vi "GET_MARKER.vi"(5 "offset":dbl, 6 "Set MKR Freq (MHz)":dbl=2000000.0 format="%#_13g", 7 "Use PK Search (T)":bool=TRUE, 8 "error in":errorcluster {"code" format="%.0x"}, 11 "Session In":refnum<visa-resource-name>="TCPIP0::169.254.70.120::inst0::INSTR") -> (0 "error out":errorcluster {"code" format="%.0x"}, 1 "Ampl_corr":dbl=-76.918, 2 "Mark Values":dbl[](array[numeric])=[40000.0232, -76.918], 3 "Session Out":refnum<visa-resource-name>="TCPIP0::169.254.70.120::inst0::INSTR")   [LabVIEW 2018]
doc: "Launches the Instrument I/O Assistant, which you can use to communicate with message-based instruments and graphically parse the response. For example you can communicate with an instrument that uses a serial, Ethernet, or GPIB interface."
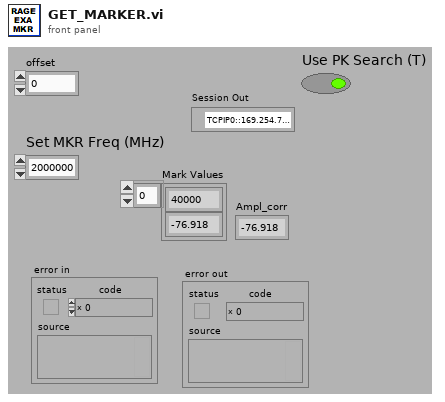
[diagram p1: front panel]
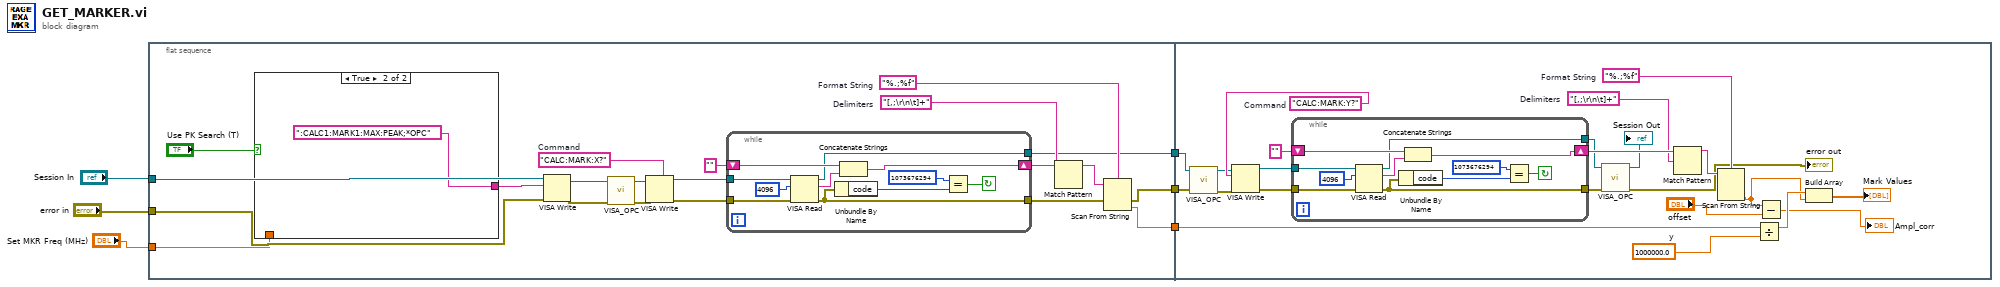
[diagram p0: block diagram]
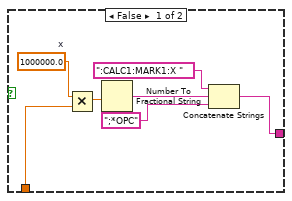
[diagram p2: hidden frame]
diagram:
  n1 = flat-sequence {
    tunnel: [w20] -> w6
    tunnel: "error in" -> [w19]
    tunnel: "Session In" -> [w18]
    tunnel: [w17] -> w4
    tunnel: [w16] -> w2
    tunnel: "Set MKR Freq (MHz)" -> [w13]
    tunnel: w6 -> [w54]
    tunnel: w4 -> [w52]
    tunnel: w2 -> [w60]
    frame #0 {
      w21 = "[,;\r\n\t]+"  # Delimiters
      w22 = "%.;%f"  # Format String
      w25 = "CALC:MARK:X?"  # Command
      n2 = case shown="True" "Use PK Search (T)" {
        tunnel: [w29 ":CALC1:MARK1:MAX:PEAK;*OPC" ("StaticText")] -> w15
        tunnel: w13 -> [w28 _]
        frame False {
          w32 = 1000000.0  # x
          n3 = Multiply(x=w32, y=w28) -> (x*y=w34:dbl)
          n4 = Number To Fractional String(number=w34) -> (F-format string=w33:string)  [unwired: 3 in]
          n5 = Concatenate Strings(":CALC1:MARK1:X " ("StaticText"), w33, ";*OPC" ("string")) -> (w29:string)
        }
        frame True {
        }
      }
      n6 = VISA Write(VISA resource name=w18, write buffer=w15, error in (no error)=w19) -> (VISA resource name out=w10:refnum<visa-resource-name>, error out=w11:errorcluster)  [unwired: 1 out]
      n7 = call "VISA_OPC.vi"("error in"=w11, "Session In"=w10) -> ("error out"=w12:errorcluster, "Session Out"=w9:refnum<visa-resource-name>)  [unwired: 7 in, 1 out]
      n8 = VISA Write(VISA resource name=w9, write buffer=w25, error in (no error)=w12) -> (VISA resource name out=w8:refnum<visa-resource-name>, error out=w7:errorcluster)  [unwired: 1 out]
      n9 = while {
        tunnel: w8 -> [w43]
        shift-right: [w37] -> w24
        shift-left: "" -> [w42]
        tunnel: w7 -> [w40]
        tunnel: [w39] -> w27
        tunnel: [w36] -> w17
        stop <- w38 continue-if-true
        n10 = VISA Read(VISA resource name=w43, byte count=u32 4096 ("byte count (0)"), error in (no error)=w40) -> (VISA resource name out=w36:refnum<visa-resource-name>, read buffer=w41:string, error out=w39:errorcluster)  [unwired: 1 out]
        n11 = Unbundle By Name(w39) -> ("code"=w45:i32)
        n12 = Concatenate Strings(w42, w41) -> (w37:string)
        n13 = Equal?(x=1073676294, y=w45) -> (x = y?=w38:bool)
      }
      n14 = Match Pattern(string=w24, regular expression=w21) -> (before substring=w23:string)  [unwired: 1 in, 3 out]
      n15 = Scan From String(format string=w22, input string=w23, error in=w27) -> (error out=w20:errorcluster, output 1=w16:dbl)  [unwired: 2 in, 2 out]
    }
    frame #1 {
      w58 = 1000000.0  # y
      w64 = "[,;\r\n\t]+"  # Delimiters
      w63 = "%.;%f"  # Format String
      w61 = "CALC:MARK:Y?"  # Command
      n16 = call "VISA_OPC.vi"("error in"=w54, "Session In"=w52) -> ("error out"=w53:errorcluster, "Session Out"=w51:refnum<visa-resource-name>)  [unwired: 7 in, 1 out]
      n17 = VISA Write(VISA resource name=w51, write buffer=w61, error in (no error)=w53) -> (VISA resource name out=w65:refnum<visa-resource-name>, error out=w66:errorcluster)  [unwired: 1 out]
      n18 = while {
        tunnel: w65 -> [w77]
        shift-right: [w71] -> w67
        shift-left: "" -> [w76]
        tunnel: w66 -> [w74]
        tunnel: [w73] -> w50
        tunnel: [w70] -> w48
        stop <- w72 continue-if-true
        n19 = VISA Read(VISA resource name=w77, byte count=u32 4096 ("byte count (0)"), error in (no error)=w74) -> (VISA resource name out=w70:refnum<visa-resource-name>, read buffer=w75:string, error out=w73:errorcluster)  [unwired: 1 out]
        n20 = Unbundle By Name(w73) -> ("code"=w79:i32)
        n21 = Concatenate Strings(w76, w75) -> (w71:string)
        n22 = Equal?(x=1073676294, y=w79) -> (x = y?=w72:bool)
      }
      n23 = call "VISA_OPC.vi"("error in"=w50, "Session In"=w48) -> ("error out"=→"error out":errorcluster, "Session Out"=→"Session Out":refnum<visa-resource-name>)  [unwired: 7 in, 1 out]
      n24 = Match Pattern(string=w67, regular expression=w64) -> (before substring=w68:string)  [unwired: 1 in, 3 out]
      n25 = Scan From String(format string=w63, input string=w68) -> (output 1=w56:dbl)  [unwired: 3 in, 3 out]
      n26 = Divide(x=w60, y=w58) -> (x/y=w59:dbl)
      n27 = Subtract(x=w56, y="offset") -> (x-y=→"Ampl_corr":dbl)
      n28 = Build Array(w59, w56) -> (→"Mark Values":dbl[])
    }
  }
